vi "Check Voltage Bounds.vi"(0 "channel configuration":T1[](array[typedef]) {"vertical offset" format="%_3p"; "vertical range" format="%_3p"}, 5 "trigger source":u8, 7 "level (V)":dbl, 11 "error in":errorcluster) -> (15 "error out":errorcluster)   [LabVIEW 2015, in "Device Session.lvclass"]
doc: "Verifies that the specified trigger voltage level is within range. This VI returns an error if <B>level</B> is outside the configured range of the <B>trigger source</B> channel.\n\n<B>Input Parameters</B>\n\n<B>channel configuration</B> is an array of the configuration of all channels configured by the 'Configure Channel' VI.\n\n<B>trigger source</B> is the channel used as the trigger source.\n\n<B>level (V)</B> specifies the voltage threshold for the trigger.\n\n<B>error in</B> describes error conditions that occur before this node runs. This input provides standard 'error in' functionality.\n\n<B>Output Parameters</B>\n\n<B>error out</B> contains error information. This output provides standard 'error out' functionality."
uses:
  Device Session.lvclass
  <instrlib>/HSAI-RIO/Types/v1/Host/Typedefs/Channel Configuration.ctl
  <instrlib>/HSAI-RIO/Types/v1/Host/Typedefs/Coupling.ctl
  <instrlib>/HSAI-RIO/Types/v1/Host/Typedefs/Impedance.ctl
  <instrlib>/HSAI-RIO/Types/v1/Host/Typedefs/Bandwidth.ctl
  <vilib>/Utility/error.llb/Error Cluster From Error Code.vi
  <vilib>/ErrorRing/Error Ring.xnode
  <instrlib>/HSAI-RIO/Types/v1/Host/niHSAI Types v1 Host.lvlib
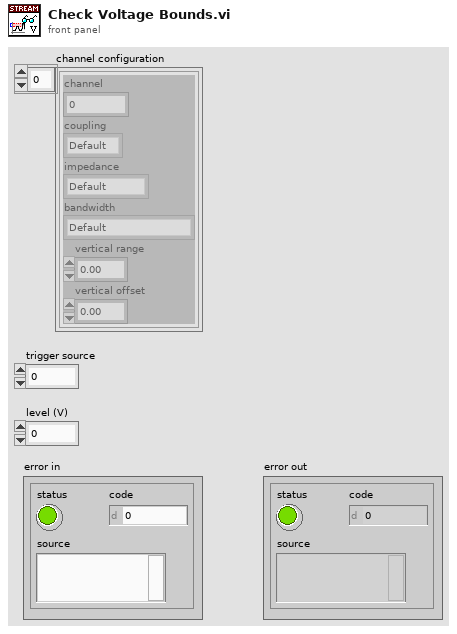
[diagram p1: front panel]
types:
  T1 = typedef "niHSAI Types v1 Host.lvlib/Channel Configuration.ctl" = cluster{"channel":u32, "coupling":T2, "impedance":T3, "bandwidth":T4, "vertical range":dbl, "vertical offset":dbl}
  T2 = typedef "niHSAI Types v1 Host.lvlib/Coupling.ctl" = enum8{"Default", "DC", "AC"}
  T3 = typedef "niHSAI Types v1 Host.lvlib/Impedance.ctl" = enum8{"Default", "1 mega ohm", "50 ohm"}
  T4 = typedef "niHSAI Types v1 Host.lvlib/Bandwidth.ctl" = enum8{"Default", "Full Bandwidth", "Anti-alias Filter"}
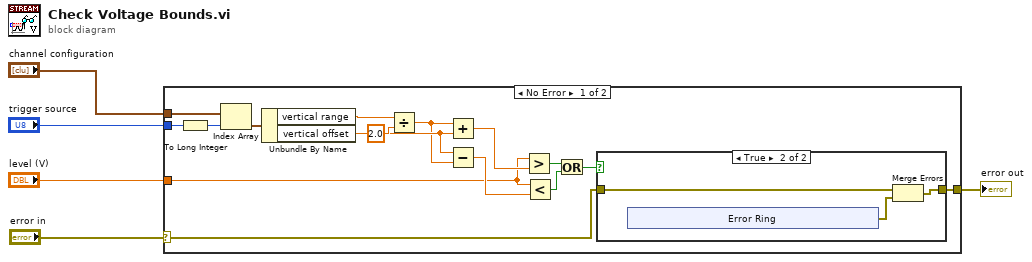
[diagram p0: block diagram]
diagram:
  n1 = case shown="No Error" "error in" {
    selector: "error in" -> [w12 w30]
    tunnel: "channel configuration" -> [w17 _]
    tunnel: "trigger source" -> [w10 _]
    tunnel: "level (V)" -> [w9 _]
    tunnel: [w13 w30] -> w1
    frame No Error {
      n2 = To Long Integer(number=w10) -> (32bit integer=w11:i32)
      n3 = Index Array(array=w17, index=w11) -> (element=w21:T1)
      n4 = Unbundle By Name(w21) -> ("vertical range"=w20:dbl, "vertical offset"=w7:dbl)
      n5 = Divide(x=w20, y=2.0 ("vertical range")) -> (x/y=w6:dbl)
      n6 = Add(x=w6, y=w7) -> (x+y=w19:dbl)
      n7 = Subtract(x=w7, y=w6) -> (x-y=w18:dbl)
      n8 = Greater?(x=w9, y=w19) -> (0:w16:bool)
      n9 = Less?(x=w9, y=w18) -> (x < y?=w15:bool)
      n10 = Or(x=w16, y=w15) -> (x .or. y?=w14:bool)
      n11 = case shown="True" w14 {
        tunnel: [w22 w25] -> w13
        tunnel: w12 -> [w22 w23]
        frame False {
        }
        frame True {
          n12 = xnode "Error Ring"() -> ("error out"=w24:errorcluster)
          n13 = Merge Errors(w23, w24) -> (w25:errorcluster)
        }
      }
    }
    frame Error {
    }
  }
  "error out" <- w1
